vi "Sum 3D to 2D.vi"(1 "3D":i32[][][](array[numeric])) -> (0 "2D":i32[][](array[numeric]))   [LabVIEW 2009]
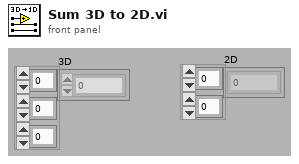
[diagram p1: front panel]
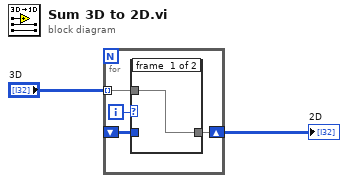
[diagram p0: block diagram]
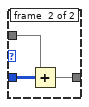
[diagram p2: hidden frame]
diagram:
  n1 = for {
    tunnel: "3D" -> [w4] mode=indexing
    shift-right: [w6] -> w1
    shift-left: _ -> [w5]
    i -> [w3]
    n2 = case shown="0" w3 {
      tunnel: [w7 w10] -> w6
      tunnel: w5 -> [_ w9]
      tunnel: w4 -> [w7 w8]
      frame #0 {
      }
      frame #1 {
        n3 = Add(x=w8, y=w9) -> (x+y=w10:i32[][])
      }
    }
  }
  "2D" <- w1
